vi "chart set style.vi"(8 "error in (no error)":errorcluster, 10 "style_id":u8, 11 "chart":u32) -> (0 "error out":errorcluster)   [LabVIEW 2015, in "xlsxwriter.lvlib"]
doc: "void chart_set_style(lxw_chart chart, uint8_t style_id);"
uses:
  xlsxwriter.lvlib
  xlsxwriter.dll
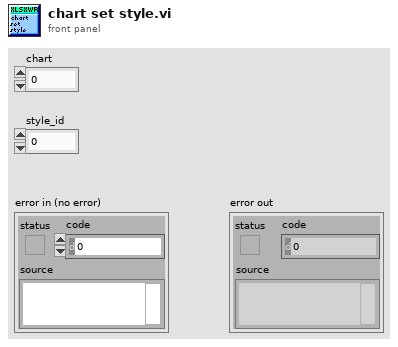
[diagram p1: front panel]
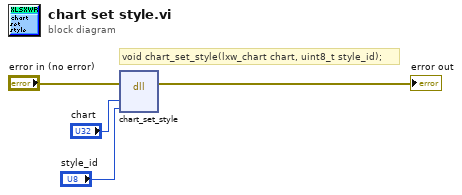
[diagram p0: block diagram]
diagram:
  # "void chart_set_style(lxw_chart chart, uint8_t style_id);"
  n1 = dll-call lib="C:/Users/WDAGUtilityAccount/Desktop/lv_vis_added_cell/xlsxwriter.*" fn="chart_set_style"(error in="error in (no error)", "chart"="chart", "style_id"="style_id") -> (error out=→"error out":errorcluster)  [unwired: 5 in, 1 out]
